vi "Re_Connection_Counter.vi"() -> ()   [LabVIEW 2012]
panel:
  in  "Re-connection counter":u32
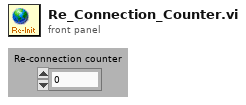
[diagram p1: front panel]
diagram:
